vi "getList.vi"(8 "error in (no error)":errorcluster, 11 "Shifters in":refnum<class "Shifters.lvclass">) -> (0 "error out":errorcluster, 2 "list":refnum<class "Shifter.lvclass">[](array[class]), 3 "Shifters out":refnum<class "Shifters.lvclass">)   [LabVIEW 2013, in "Shifters.lvclass"]
uses:
  Shifters.lvclass
  Shifter.lvclass
  Shifters.lvclass/Shifters.ctl
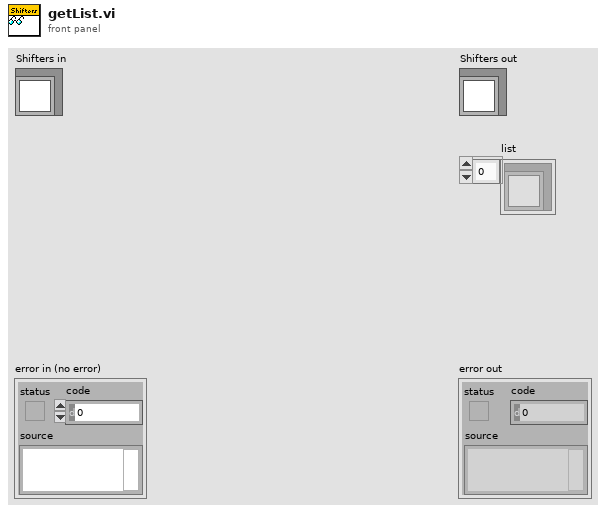
[diagram p1: front panel]
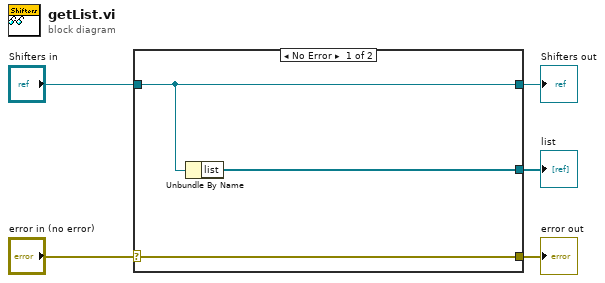
[diagram p0: block diagram]
diagram:
  n1 = case shown="No Error" "error in (no error)" {
    selector: "error in (no error)" -> [w8 w9]
    tunnel: [w8 w9] -> w4
    tunnel: [w7 w10] -> w2
    tunnel: "Shifters in" -> [w7 w10]
    tunnel: [w6 _] -> w1
    frame No Error {
      n2 = Unbundle By Name(w7) -> ("list"=w6:refnum<class "Shifter.lvclass">[])
    }
    frame Error {
    }
  }
  "error out" <- w4
  "Shifters out" <- w2
  "list" <- w1
